vi "ziPollDataEx.vi"(8 "error in":errorcluster, 10 "Timeout ms (50)":i32=50, 11 "Handle In":T1 {"Handle" format="0x%08x"; "Conn" format="0x%08x"}) -> (0 "error out":errorcluster, 1 "Timestamp (ticks)":u64=2149, 2 "PathArray":string[](array[string]), 3 "Handle Out":T1 {"Handle" format="0x%08x"; "Conn" format="0x%08x"}, 4 "Value Double":dbl, 5 "Timed Out":bool, 6 "Value Int":i32, 7 "ziValueType":T2)   [LabVIEW 2009, in "Zurich Instruments LabOne.lvlib"]
doc: "Use this vi to receive all value changes that occur in nodes that have been subscribed to, or in children of nodes that have been subscribed to. This vi returns immediately if data is pending. Otherwise it waits for data for up to <b>Timeout</b> milliseconds before it returns with <b>Timed Out</b> true. When no data event was received within <b>TimeOut</b> milliseconds, <b>ziValueType</b> will be NONE and the <b>Timed Out</b> will be true. \nIf the <b>ziValueType</b> is INTEGER_DATA or DOUBLE_DATA, the data can be retrieved from <b>Value Int</b> and <b>Value Double</b> connectors. For all other value types, use ziGetEvent.vi to retrieve the appropriate data from the handle."
uses:
  <instrlib>/Zurich Instruments LabOne/Zurich Instruments LabOne.lvlib
  <instrlib>/Zurich Instruments LabOne/Public/Data/ziTypePollType.ctl
  <instrlib>/Zurich Instruments LabOne/Public/ziTypeHandle.ctl
  <instrlib>/Zurich Instruments LabOne/Private/ziLV64.dll
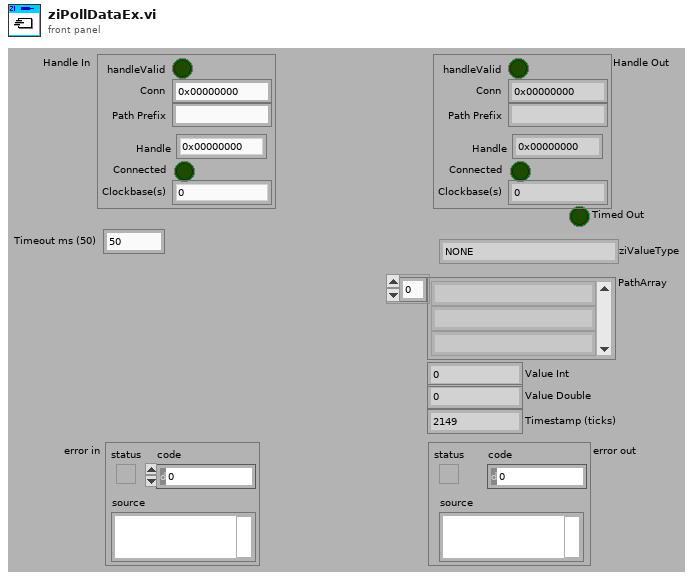
[diagram p1: front panel]
types:
  T1 = typedef "Zurich Instruments LabOne.lvlib/ziTypeHandle.ctl" = cluster{"handleValid":bool, "Conn":u64, "Path Prefix":string, "Handle":u64, "Connected":bool, "Clockbase(s)":dbl}
  T2 = typedef "Zurich Instruments LabOne.lvlib/ziTypePollType.ctl" = enum16{"NONE", "DOUBLE_DATA", "INTEGER_DATA", "DEMOD_SAMPLE", "SCOPE_WAVE_HF2", "AUXIN_SAMPLE", "DIO_SAMPLE", "BYTE_ARRAY", "PWA_WAVE", "9", "10", "11", "12", "13", "14", "15", "TREE_CHANGE_DEPRI", "17", "ERROR", "19", "20", "21", "22", "23", "24", "25", "26", "27", "28", "29", "30", "31", "DOUBLE_DATA_TS", "INTEGER_DATA_TS", "34", "SCOPE_WAVE", "SCOPE_WAVE_EX", "37", "BYTE_ARRAY_TS", "39", "40", "41", "42", "43", "44", "45", "CNT_DATA", "47", "TREE_CHANGE", "49", "50", "51", "52", "53", "54", "55", "56", "57", "58", "59", "60", "61", "62", "63", "SWEEPER_DATA", "SPECTRUM_DATA", "ADVISOR_DATA", "VECTOR_DATA", "IMP_DATA", "SHF_GENERATOR_WAVEFORM_DATA", "SHF_RESULT_LOGGER_DATA", "SHF_SCOPE_DATA", "SHF_DEMOD_DATA"}
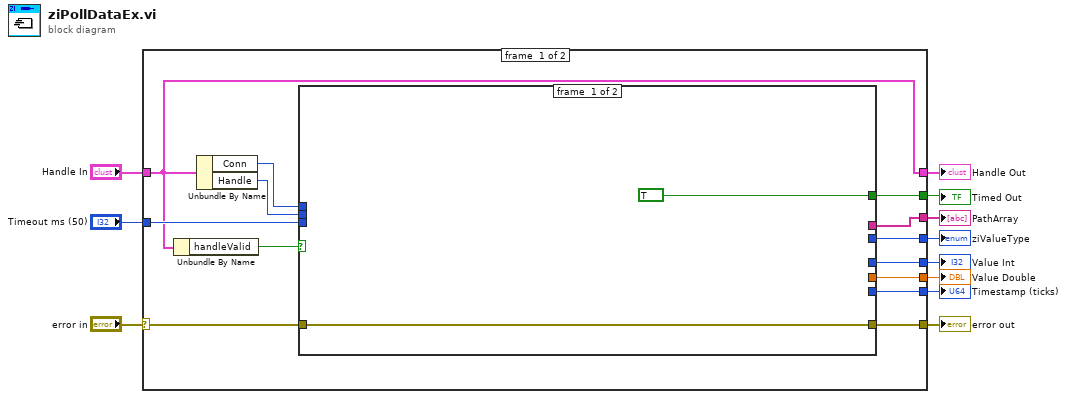
[diagram p0: block diagram]
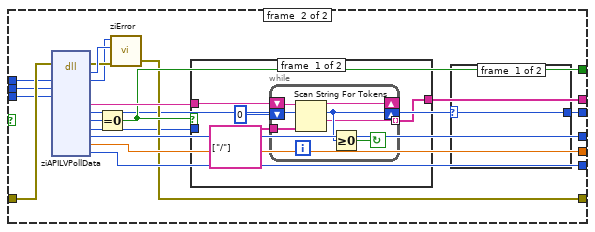
[diagram p2: hidden frame]
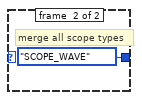
[diagram p3: hidden frame]
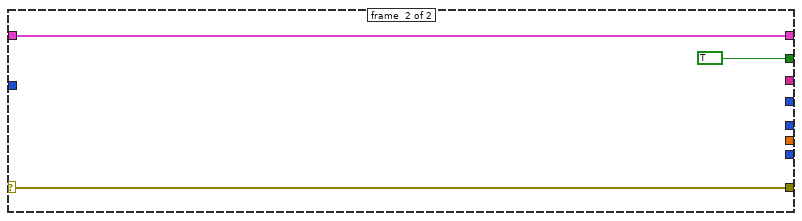
[diagram p5: hidden frame]
diagram:
  n1 = case shown="No Error" "error in" {
    selector: "error in" -> [w17 w59]
    tunnel: [w24 w59] -> w11
    tunnel: "Timeout ms (50)" -> [w23 _]
    tunnel: [w22 _] -> w9
    tunnel: [w21 TRUE] -> w8
    tunnel: [w20 _] -> w7
    tunnel: [w19 _] -> w6
    tunnel: [w18 _] -> w5
    tunnel: "Handle In" -> [w12 w60]
    tunnel: [w12 w60] -> w3
    tunnel: [w15 _] -> w1
    frame #0 {
      n2 = Unbundle By Name(w12) -> ("handleValid"=w16:bool)
      n3 = Unbundle By Name(w12) -> ("Conn"=w14:u64, "Handle"=w13:u64)
      n4 = case shown="True" w16 {
        tunnel: w17 -> [w26 w42]
        tunnel: w14 -> [_ w41]
        tunnel: [w26 w31] -> w24
        tunnel: [_ w34] -> w22
        tunnel: w13 -> [_ w40]
        tunnel: [_ w27] -> w15
        tunnel: [_ w38] -> w20
        tunnel: [_ w39] -> w19
        tunnel: w23 -> [_ w37]
        tunnel: [TRUE w35] -> w21
        tunnel: [_ w33] -> w18
        frame #0 {
        }
        frame #1 {
          n5 = dll-call lib="C:/Program Files/National Instruments/LabVIEW 2009/instr.lib/Zurich Instruments LabOne/Private/ziLV*.*" fn="ziAPILVPollData"(error in=w42, "Conn"=w41, "ziEventBuffer"=w40, "TimeOut(ms)"=w37) -> (error out=w43:errorcluster, "return type"=w44:u32, "Conn"=w29:u64, "Path"=w36:string, "Type"=w28:u32, "Count"=w32:i32, "Offset"=w30:i32, "int"=w38:i32, "double"=w39:dbl, "timestamp"=w33:u64)  [unwired: 6 in, 6 out]
          n6 = Equal To 0?(x=w32) -> (x = 0?=w35:bool)
          n7 = call <instrlib>:"ziError.vi"("Conn"=w29, "ziErrorCode"=w44, "Error In"=w43) -> ("Error Out"=w31:errorcluster)  [unwired: 2 in, 1 out]
          n8 = case shown="False" w35 {
            tunnel: w36 -> [w48 _]
            tunnel: [w49 _] -> w34
            tunnel: w30 -> [_ _]
            frame #0 {
              n9 = while {
                shift-right: [w55] -> _
                shift-left: w48 -> [w57]
                shift-right: [w54] -> _
                shift-left: 0 ("offset past token") -> [w56]
                tunnel: [w52] -> w49 mode=indexing
                tunnel: string[] ["/"] ("delimiters (\\s,\\t,\\r,\\n)") -> [w51]
                stop <- w53 continue-if-true
                n10 = Scan String For Tokens(6:w51, 8:w56, 9:w57) -> (1:w52:string, 2:w54:i32, 3:w55:string)  [unwired: 1 in, 3 out]
                n11 = Greater Or Equal To 0?(x=w54) -> (x >= 0?=w53:bool)
              }
            }
            frame #1 {
            }
          }
          n12 = case shown="4, 36" w28 {
            selector: w28 -> [w45 _]
            tunnel: [w45 ziTypePollType."SCOPE_WAVE" ("ziValueType")] -> w27
            frame #0 {
            }
            frame #1 {
              # "merge all scope types"
            }
          }
        }
      }
    }
    frame #1 {
    }
  }
  "error out" <- w11
  "ziValueType" <- w1
  "Timed Out" <- w8
  "Handle Out" <- w3
  "PathArray" <- w9
  "Value Double" <- w6
  "Value Int" <- w7
  "Timestamp (ticks)" <- w5
